vi "Mittelwertbildung.vi"(9 "Anzahl Werte":u8, 11 "Neuer Wert":sgl) -> (0 "Array":sgl[](array[numeric]), 2 "gemittelter Wert":sgl, 3 "Wert":sgl)   [LabVIEW 2020, in "Allgemein.lvlib"]
uses:
  Allgemein.lvlib
panel:
  # "Ablaufinvariante Ausführung"
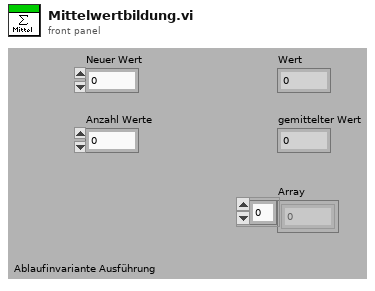
[diagram p1: front panel]
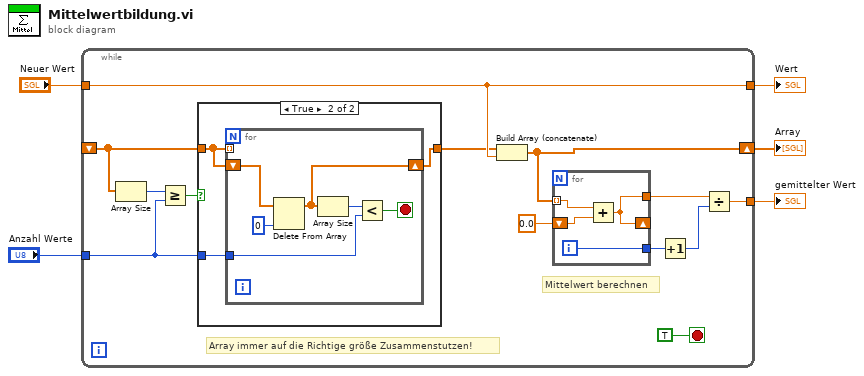
[diagram p0: block diagram]
diagram:
  n1 = while {
    shift-right: [w17] -> w1
    shift-left: _ -> [w9]
    tunnel: "Neuer Wert" -> [w10]
    tunnel: "Anzahl Werte" -> [w6]
    tunnel: [w12] -> w3
    tunnel: [w10] -> w2
    stop <- TRUE stop-if-true
    # "Mittelwert berechnen"
    # "Array immer auf die Richtige größe Zusammenstutzen!"
    n2 = Array Size(array=w9) -> (size(s)=w11:i32)
    n3 = Greater Or Equal?(x=w11, y=w6) -> (x >= y?=w7:bool)
    n4 = case shown="True" w7 {
      tunnel: w9 -> [w19 w21]
      tunnel: [w19 w20] -> w8
      tunnel: w6 -> [_ w22]
      frame False {
      }
      frame True {
        n5 = for {
          tunnel: w22 -> [w26]
          tunnel: w21 -> [_] mode=indexing
          shift-right: [w23] -> w20
          shift-left: w21 -> [w28]
          stop <- w25 stop-if-true
          n6 = Delete From Array(array=w28, index=0 ("Index")) -> (array with subset deleted=w23:sgl[])  [unwired: 1 in, 1 out]
          n7 = Array Size(array=w23) -> (size(s)=w27:i32)
          n8 = Less?(x=w27, y=w26) -> (x < y?=w25:bool)
        }
      }
    }
    n9 = Build Array (concatenate)(w8, w10) -> (w17:sgl[])
    n10 = for {
      tunnel: w17 -> [w32] mode=indexing
      shift-right: [w30] -> _
      shift-left: sgl 0.0 ("Neuer Wert") -> [w31]
      tunnel: [w30] -> w14
      tunnel: [w29] -> w15
      i -> [w29]
      n11 = Add(x=w32, y=w31) -> (x+y=w30:sgl)
    }
    n12 = Increment(x=w15) -> (x+1=w13:i32)
    n13 = Divide(x=w14, y=w13) -> (x/y=w12:sgl)
  }
  "Wert" <- w2
  "gemittelter Wert" <- w3
  "Array" <- w1
